vi "App Closing.vi"(8 "erro":errorcluster) -> (0 "error out":errorcluster)   [LabVIEW 2014]
panel:
  # "Application is closing ..."
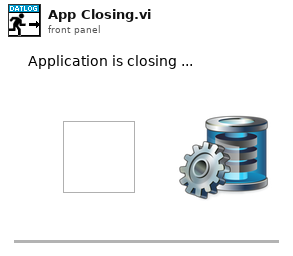
[diagram p1: front panel]
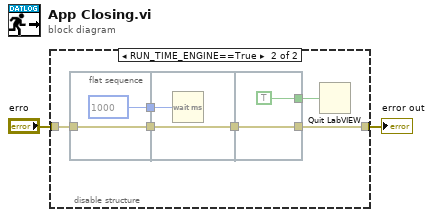
[diagram p0: block diagram]
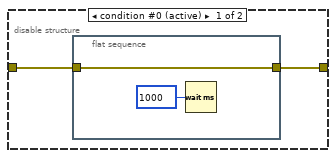
[diagram p2: hidden frame]
diagram:
  n1 = disable-structure shown="RUN_TIME_ENGINE==True" {
    disable-tunnel: [w4 w9] -> w2
    disable-tunnel: "erro" -> [w3 w11]
    frame condition #0 (active) {
      n2 = flat-sequence {
        tunnel: [w6] -> w4
        tunnel: w3 -> [w6]
        frame #0 {
          n3 = Wait (ms)(milliseconds to wait=u32 1000) -> ()  [unwired: 1 out]
        }
      }
    }
    frame condition #1 {
      n4 = flat-sequence {
        tunnel: [u32 1000 ("milliseconds to wait")] -> w12
        tunnel: w11 -> [w13]
        tunnel: [w13] -> w10
        tunnel: w12 -> [w16]
        tunnel: w10 -> [w15]
        tunnel: [w15] -> w8
        tunnel: [w18] -> w9
        tunnel: w8 -> [w18]
        tunnel: [TRUE] -> w7
        frame #0 {
        }
        frame #1 {
          n5 = Wait (ms)(milliseconds to wait=w16) -> ()  [unwired: 1 out]
        }
        frame #2 {
        }
      }
      n6 = Quit LabVIEW(quit? (T)=w7) -> ()
    }
  }
  "error out" <- w2
